vi "exnSharedSub locale global.vi"() -> ()   [LabVIEW 2020]
panel:
  in  "config header text":string="This Express VI is configured as follows:"
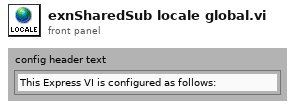
[diagram p1: front panel]
diagram:
